vi "send TRA command-v-03.vi"(11 "command":string) -> ()   [LabVIEW 2011]
panel:
  out "error out":errorcluster
  out "motor number":i32
  out "axis number":i32
  out "Mirror number":i32
  out "decimal integer string":string
  out "number in cluster":u16
  out "Mirror information":T1
  in  "Mirror information Array":T2(array[cluster])=[{"Motor number"=0, "Mirror name"="TA2", "Axis"="horizontal", "DS command address"="dstp://192.168.11.36/Capillary_100PP_1_command", "DS status address"="dstp://192.168.11.36/Capillary_100PP_1_status"}, {"Motor number"=1, "Mirror name"="TA2", "Axis"="vertical", "DS command address"="dstp://192.168.11.36/Capillary_100PP_1_command", "DS status address"="dstp://192.168.11.36/Capillary_100PP_1_status"}, {"Motor number"=2, "Mirror name"="", "Axis"="", "DS command address"="dstp://192.168.11.36/Capillary_100PP_1_command", "DS status address"="dstp://192.168.11.36/Capillary_100PP_1_status"}, {"Motor number"=3, "Mirror name"="", "Axis"="", "DS command address"="dstp://192.168.11.36/Capillary_100PP_1_command", "DS status address"="dstp://192.168.11.36/Capillary_100PP_1_status"}, {"Motor number"=4, "Mirror name"="", "Axis"="", "DS command address"="dstp://192.168.11.36/Capillary_100PP_1_command", "DS status address"="dstp://192.168.11.36/Capillary_100PP_1_status"}, {"Motor number"=5, "Mirror name"="M23", "Axis"="", "DS command address"="dstp://192.168.11.36/Capillary_100PP_1_command", "DS status address"="dstp://192.168.11.36/Capillary_100PP_1_status"}, {"Motor number"=6, "Mirror name"="M23", "Axis"="", "DS command address"="dstp://192.168.11.36/Capillary_100PP_1_command", "DS status address"="dstp://192.168.11.36/Capillary_100PP_1_status"}, {"Motor number"=7, "Mirror name"="OAP", "Axis"="", "DS command address"="dstp://192.168.11.36/Capillary_100PP_2_command", "DS status address"="dstp://192.168.11.36/Capillary_100PP_2_status"}, {"Motor number"=8, "Mirror name"="OAP", "Axis"="", "DS command address"="dstp://192.168.11.36/Capillary_100PP_2_command", "DS status address"="dstp://192.168.11.36/Capillary_100PP_2_status"}]
  out "#loops ds read":i32
  out "In range?":bool
  in  "Actual status_1 3":string="dstp://192.168.11.36/Capillary_100PP_1_status"
  in  "Target_1 3":string="dstp://192.168.11.36/Capillary_100PP_1_command"
  out "Step size":sgl=0.001 caption="Step Size  (mm)" format="%#_6f"
  out "Motor Positions Actual":T3={"1.43938", "3.20284", "5.06802", "3.66263", "4.85177", "4.42890", "000033", "000033", "000033", "000033", "000033", "000033"}
  out "Status":string="Calculating new motor position"
  in  "Target Motor Positions":T4={"1.43938", "3.20284", "5.06802", "3.66263", "4.85177", "4.42890", FALSE, FALSE, FALSE, FALSE, FALSE, FALSE}
  out "Mirror number":u16=1
  out "APulses":u16=300
  out "aDir":bool=TRUE
  # "go:5000:cw:01"
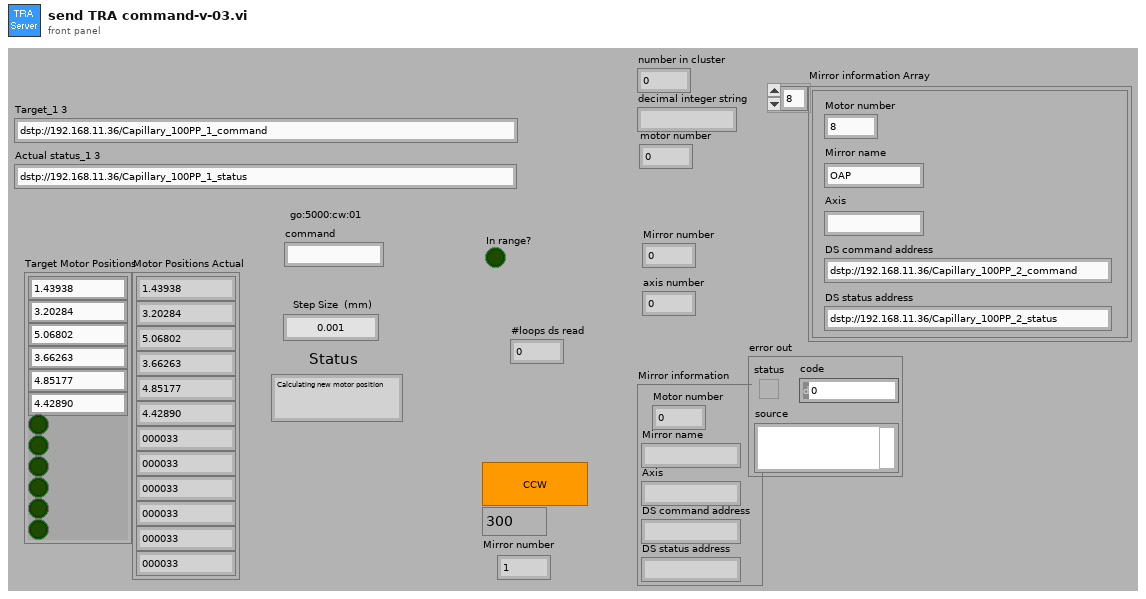
[diagram p1: front panel]
types:
  T1 = cluster{"Motor number":u16, "Mirror name":string, "Axis":string, "DS command address":string, "DS status address":string}
  T2 = cluster{"Motor number":u16, "Mirror name":string, "Axis":string, "DS command address":string, "DS status address":string}[]
  T3 = cluster{string, string, string, string, string, string, string, string, string, string, string, string}
  T4 = cluster{string, string, string, string, string, string, bool, bool, bool, bool, bool, bool}
  T5 = enum16{"Read", "Write", "ReadWrite", "BufferedRead", "BufferedReadWrite"}
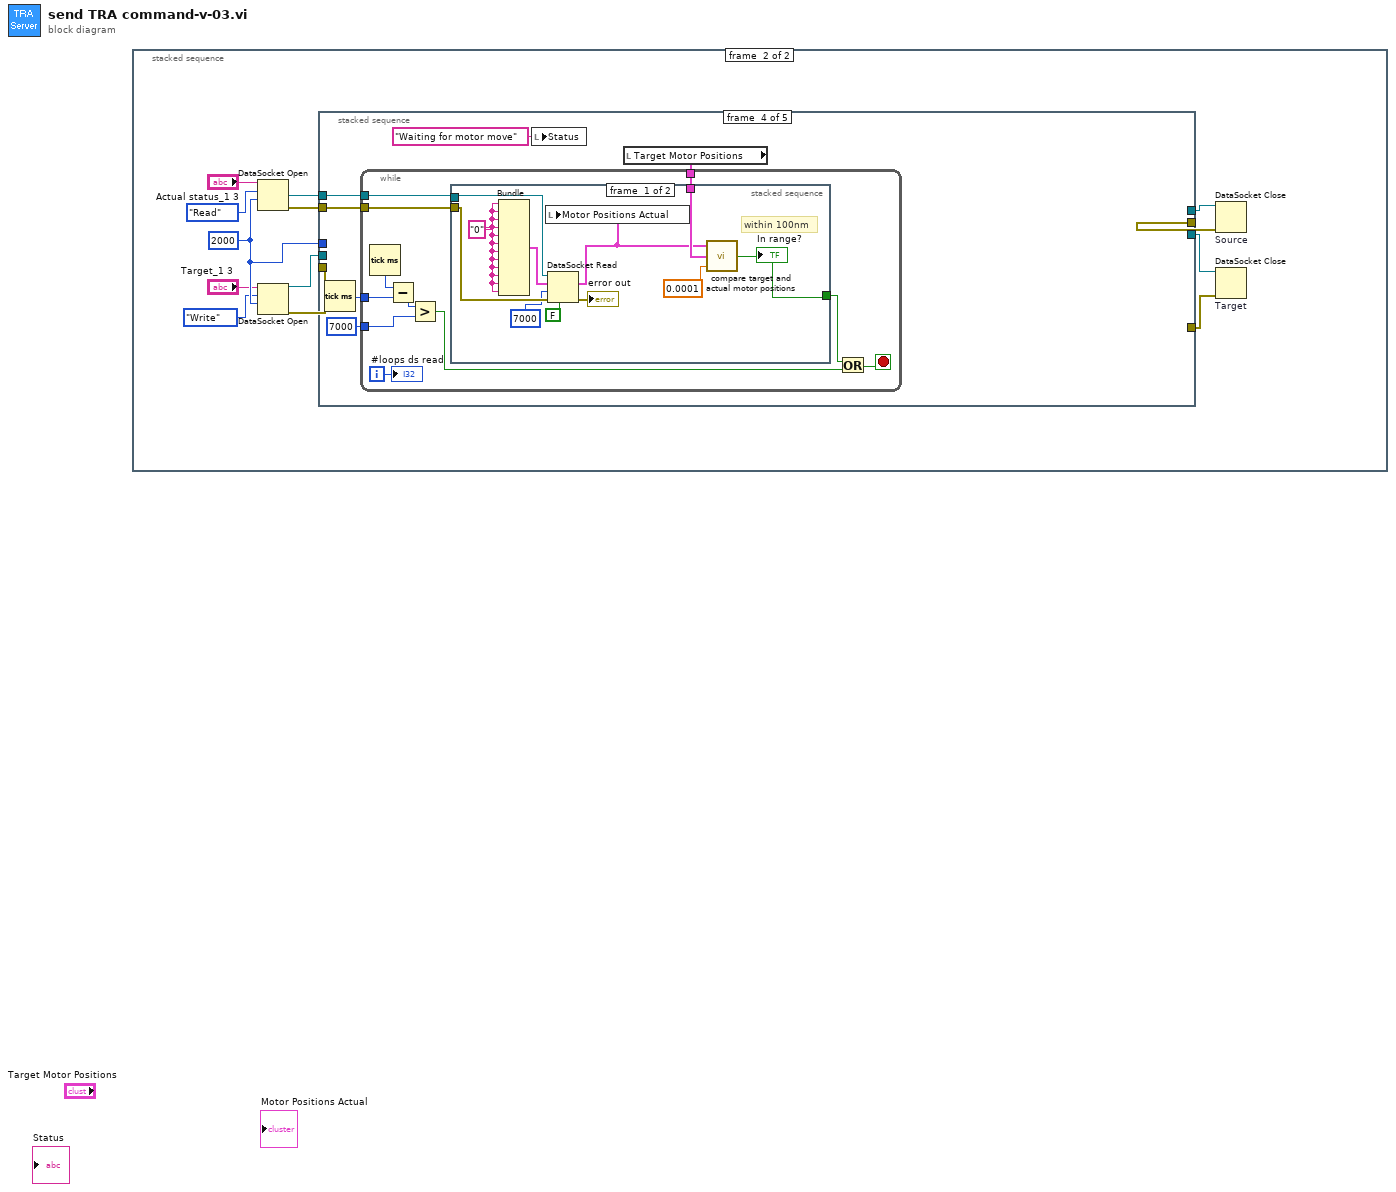
[diagram p0: block diagram]
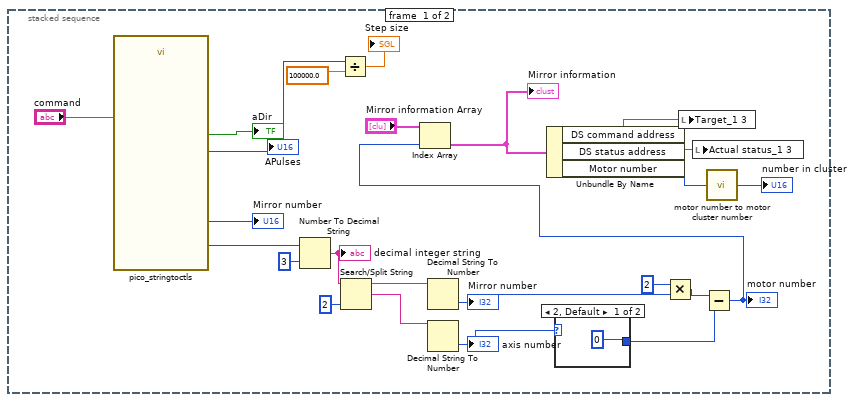
[diagram p2: hidden frame]
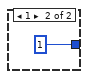
[diagram p3: hidden frame]
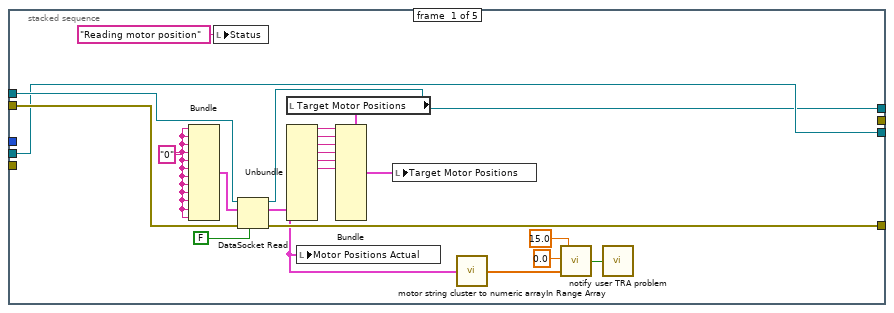
[diagram p4: hidden frame]
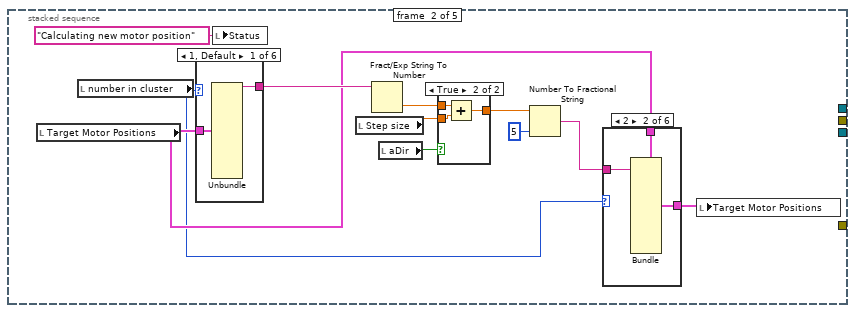
[diagram p5: hidden frame]
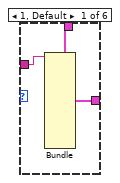
[diagram p6: hidden frame]
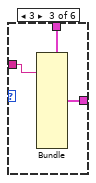
[diagram p7: hidden frame]
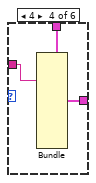
[diagram p8: hidden frame]
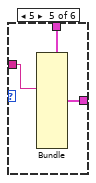
[diagram p9: hidden frame]
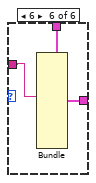
[diagram p10: hidden frame]
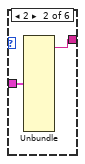
[diagram p11: hidden frame]
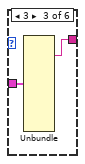
[diagram p12: hidden frame]
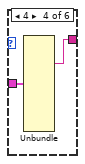
[diagram p13: hidden frame]
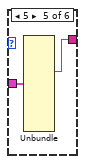
[diagram p14: hidden frame]
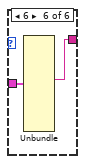
[diagram p15: hidden frame]
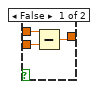
[diagram p16: hidden frame]
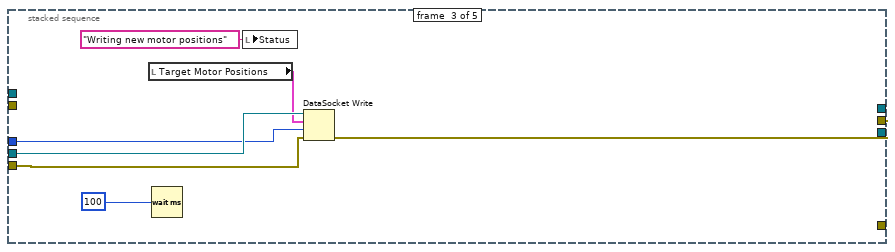
[diagram p17: hidden frame]
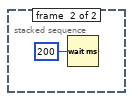
[diagram p18: hidden frame]
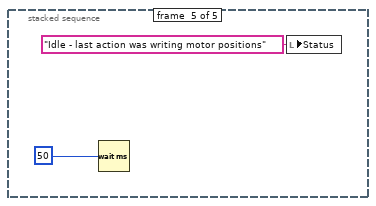
[diagram p19: hidden frame]
diagram:
  n1 = stacked-sequence {
    frame #0 {
      n2 = call "pico_stringtoctls.vi"("String in"="command") -> ("aDir"=→"aDir":bool, "APulses"=w19:u16, "MIRROR"=w12:u16)  [unwired: 7 out]
      "APulses" <- w19
      "Mirror number" <- w12
      n3 = Number To Decimal String(number=w12, width (-)=i16 3) -> (decimal integer string=w10:string)
      "decimal integer string" <- w10
      n4 = Divide(x=w19, y=100000.0) -> (x/y=→"Step size":dbl)
      n5 = Search/Split String(string=w10, offset (0)=2) -> (substring before match=w8:string, match + rest of string=w7:string)  [unwired: 1 in, 1 out]
      n6 = Decimal String To Number(string=w8) -> (number=w5:i32)  [unwired: 2 in, 1 out]
      "Mirror number" <- w5
      n7 = Decimal String To Number(string=w7) -> (number=w6:i32)  [unwired: 2 in, 1 out]
      "axis number" <- w6
      n8 = case shown="2, Default" w6 {
        tunnel: [0 ("x") 1 ("axis number")] -> w2
        frame 2, Default {
        }
        frame 1 {
        }
      }
      n9 = Multiply(x=2, y=w5) -> (x*y=w3:i32)
      n10 = Subtract(x=w3, y=w2) -> (x-y=w1:i32)
      "motor number" <- w1
      n11 = Index Array(array="Mirror information Array", index=w1) -> (element=w14:T1)
      "Mirror information" <- w14
      n12 = Unbundle By Name(w14) -> ("DS command address"=w17:string, "DS status address"=w16:string, "Motor number"=w13:u16)
      n13 = local write "Target_1 3"(w17) -> ()
      n14 = local write "Actual status_1 3"(w16) -> ()
      n15 = call "motor number to motor cluster number.vi"("Motor number"=w13) -> ("number in cluster"=→"number in cluster":u16)
    }
    frame #1 {
      w32 = 2000 ("ms timeout (10000)")
      n16 = DataSocket Open(9:w32, 10:T5."Read" ("mode"), 11:"Actual status_1 3") -> (0:w33:errorcluster, 3:w30:refnum<k13>)  [unwired: 1 in]
      n17 = DataSocket Open(9:w32, 10:T5."Write" ("mode"), 11:"Target_1 3") -> (0:w34:errorcluster, 3:w31:refnum<k13>)  [unwired: 1 in]
      n18 = stacked-sequence {
        tunnel: w31 -> [w45 _ w113 _ _]
        tunnel: w32 -> [_ _ w112 _ _]
        tunnel: w34 -> [_ _ w111 _ _]
        tunnel: [w44 _ _ _ _] -> w35
        tunnel: [_ _ w114 _ _] -> w36
        tunnel: w30 -> [w57 _ _ w120 _]
        tunnel: w33 -> [w56 _ _ w119 _]
        tunnel: [w45 _ _ _ _] -> w37
        tunnel: [w55 _ _ _ _] -> w38
        frame #0 {
          w58 = "0"
          n19 = Bundle(w58, w58, w58, w58, w58, w58, w58, w58, w58, w58, w58, w58) -> (w59:T3)  [unwired: 1 out]
          n20 = local write "Status"("Reading motor position" ("Status")) -> ()
          n21 = DataSocket Read(6:FALSE ("wait?"), 8:w56, 10:w59, 11:w57) -> (0:w55:errorcluster, 2:w43:T3, 3:w44:refnum<k13>)  [unwired: 5 out]
          n22 = local read "Target Motor Positions"() -> (w54:T4)
          n23 = Unbundle(w43) -> (w52:string, w51:string, w50:string, w49:string, w48:string, w47:string)  [unwired: 6 out]
          n24 = local write "Motor Positions Actual"(w43) -> ()
          n25 = Bundle(cluster=w54, w52, w51, w50, w49, w48, w47) -> (w53:T4)  [unwired: 6 out]
          n26 = local write "Target Motor Positions"(w53) -> ()
          n27 = call "motor string cluster to numeric array.vi"("Motor Positions Actual"=w43) -> ("Array"=w42:dbl[])
          n28 = call "In Range Array.vi"("Array"=w42, "lower limit"=0.0, "upper limit"=15.0) -> ("At least 1 out of range"=w39:bool)
          n29 = call "notify user TRA problem.vi"("At least 1 out of range"=w39) -> ()
        }
        frame #1 {
          n30 = local read "Target Motor Positions"() -> (w63:T4)
          n31 = local read "number in cluster"() -> (w62:u16)
          n32 = case shown="1, Default" w62 {
            tunnel: w63 -> [w91 w93 w95 w97 w99 w101]
            tunnel: [w90 w92 w94 w96 w98 w100] -> w68
            frame 1, Default {
              n33 = Unbundle(w91) -> (w90:string)  [unwired: 11 out]
            }
            frame 2 {
              n34 = Unbundle(w93) -> (w92:string)  [unwired: 11 out]
            }
            frame 3 {
              n35 = Unbundle(w95) -> (w94:string)  [unwired: 11 out]
            }
            frame 4 {
              n36 = Unbundle(w97) -> (w96:string)  [unwired: 11 out]
            }
            frame 5 {
              n37 = Unbundle(w99) -> (w98:string)  [unwired: 11 out]
            }
            frame 6 {
              n38 = Unbundle(w101) -> (w100:string)  [unwired: 11 out]
            }
          }
          n39 = local write "Status"("Calculating new motor position" ("Status")) -> ()
          n40 = local read "Step size"() -> (w66:sgl)
          n41 = Fract/Exp String To Number(string=w68) -> (number=w65:dbl)  [unwired: 4 out]
          n42 = local read "aDir"() -> (w67:bool)
          n43 = case shown="True" w67 {
            tunnel: [w102 w107] -> w64
            tunnel: w65 -> [w104 w106]
            tunnel: w66 -> [w103 w105]
            frame False {
              n44 = Subtract(x=w104, y=w103) -> (x-y=w102:dbl)
            }
            frame True {
              n45 = Add(x=w106, y=w105) -> (x+y=w107:dbl)
            }
          }
          n46 = Number To Fractional String(number=w64, precision (6)=i16 5) -> (F-format string=w69:string)  [unwired: 2 out]
          n47 = case shown="2" w62 {
            tunnel: w63 -> [w73 w77 w80 w83 w86 w89]
            tunnel: w69 -> [w74 w76 w79 w82 w85 w88]
            tunnel: [w72 w75 w78 w81 w84 w87] -> w70
            frame 1, Default {
              n48 = Bundle(cluster=w73, w74) -> (w72:T4)  [unwired: 11 out]
            }
            frame 2 {
              n49 = Bundle(cluster=w77, w76) -> (w75:T4)  [unwired: 11 out]
            }
            frame 3 {
              n50 = Bundle(cluster=w80, w79) -> (w78:T4)  [unwired: 11 out]
            }
            frame 4 {
              n51 = Bundle(cluster=w83, w82) -> (w81:T4)  [unwired: 11 out]
            }
            frame 5 {
              n52 = Bundle(cluster=w86, w85) -> (w84:T4)  [unwired: 11 out]
            }
            frame 6 {
              n53 = Bundle(cluster=w89, w88) -> (w87:T4)  [unwired: 11 out]
            }
          }
          n54 = local write "Target Motor Positions"(w70) -> ()
        }
        frame #2 {
          n55 = local read "Target Motor Positions"() -> (w109:T4)
          n56 = Wait (ms)(milliseconds to wait=u32 100) -> ()  [unwired: 1 out]
          n57 = local write "Status"("Writing new motor positions" ("Status")) -> ()
          n58 = DataSocket Write(8:w111, 9:w112, 10:w109, 11:w113) -> (0:w114:errorcluster)  [unwired: 2 out]
        }
        frame #3 {
          n59 = Tick Count (ms)() -> (millisecond timer value=w116:u32)
          n60 = local write "Status"("Waiting for motor move" ("Status")) -> ()
          n61 = local read "Target Motor Positions"() -> (w117:T4)
          n62 = while {
            tunnel: w120 -> [w131]
            tunnel: w119 -> [w130]
            tunnel: w117 -> [w128]
            tunnel: w116 -> [w125]
            tunnel: u32 7000 ("y") -> [w123]
            i -> [w127]
            stop <- w122 stop-if-true
            n63 = Tick Count (ms)() -> (millisecond timer value=w126:u32)
            n64 = Subtract(x=w126, y=w125) -> (x-y=w124:u32)
            n65 = Greater?(x=w124, y=w123) -> (0:w121:bool)
            n66 = stacked-sequence {
              tunnel: w131 -> [w139 _]
              tunnel: w130 -> [w138 _]
              tunnel: [w135 _] -> w129
              tunnel: w128 -> [w134 _]
              frame #0 {
                w140 = "0"
                # "within 100nm"
                n67 = Bundle(w140, w140, w140, w140, w140, w140, w140, w140, w140, w140, w140, w140) -> (w141:T3)  [unwired: 1 out]
                n68 = DataSocket Read(6:FALSE ("wait?"), 8:w138, 9:7000 ("ms timeout (10000)"), 10:w141, 11:w139) -> (0:→"error out":errorcluster, 2:w133:T3)  [unwired: 5 out]
                n69 = local write "Motor Positions Actual"(w133) -> ()
                n70 = call "compare target and actual motor positions.vi"("y"=0.0001, "Target Motor Positions"=w134, "Motor Positions Actual"=w133) -> ("Boolean"=w135:bool)
                "In range?" <- w135
              }
              frame #1 {
                n71 = Wait (ms)(milliseconds to wait=u32 200) -> ()  [unwired: 1 out]
              }
            }
            n72 = Or(x=w129, y=w121) -> (x .or. y?=w122:bool)
            "#loops ds read" <- w127
          }
        }
        frame #4 {
          n73 = Wait (ms)(milliseconds to wait=u32 50) -> ()  [unwired: 1 out]
          n74 = local write "Status"("Idle - last action was writing motor positions" ("Status")) -> ()
        }
      }
      n75 = DataSocket Close "Source"(8:w36, 11:w35) -> ()  [unwired: 3 out]
      n76 = DataSocket Close "Target"(8:w38, 11:w37) -> ()  [unwired: 3 out]
    }
  }
